vi "Heat Up Macro Find Small Flow Index.vi"(6 "Gallons":string[](array[string]), 8 "Error In":errorcluster, 9 "Draw Flag Column":string[](array[string]), 10 "Elapsed Time":string[](array[string]), 11 "Gallon Target":dbl) -> (0 "Error Out":errorcluster, 1 "Gallons":dbl, 2 "Time":dbl, 3 "Error Array. If all false":bool[](array[boolean]), 4 "Numeric":i32)   [LabVIEW 2019]
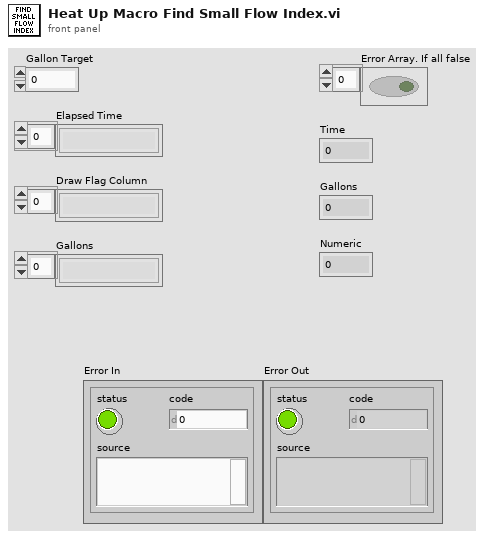
[diagram p1: front panel]
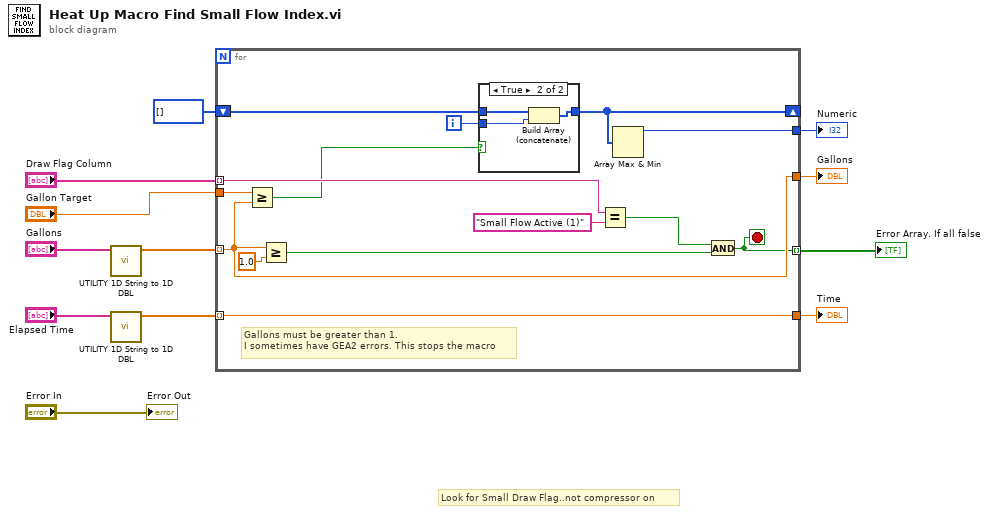
[diagram p0: block diagram]
diagram:
  # "Look for Small Draw Flag..not compressor on"
  n1 = call "UTILITY 1D String to 1D DBL.vi"("Save Data"="Gallons") -> ("DBL"=w3:dbl[])  [unwired: 10 in]
  n2 = call "UTILITY 1D String to 1D DBL.vi"("Save Data"="Elapsed Time") -> ("DBL"=w6:dbl[])  [unwired: 10 in]
  n3 = for {
    tunnel: w3 -> [w17] mode=indexing
    tunnel: [w17] -> w4
    tunnel: w6 -> [w26] mode=indexing
    tunnel: [w26] -> w9
    tunnel: "Gallon Target" -> [w25]
    shift-right: [w23] -> _
    shift-left: i32[] [] -> [w24]
    tunnel: [w22] -> w12
    tunnel: "Draw Flag Column" -> [w20] mode=indexing
    tunnel: [w13] -> w11 mode=indexing
    i -> [w21]
    stop <- w13 stop-if-true
    # "Gallons must be greater than 1.\nI sometimes have GEA2 errors. This stops the macro"
    n4 = Greater Or Equal?(x=w25, y=w17) -> (x >= y?=w18:bool)
    n5 = Greater Or Equal?(x=w17, y=1.0) -> (x >= y?=w14:bool)
    n6 = case shown="True" w18 {
      tunnel: w24 -> [w27 w30]
      tunnel: [w27 w29] -> w23
      tunnel: w21 -> [_ w28]
      frame False {
      }
      frame True {
        n7 = Build Array (concatenate)(w30, w28) -> (w29:i32[])
      }
    }
    n8 = Equal?(x=w20, y="Small Flow Active (1)") -> (x = y?=w15:bool)
    n9 = Array Max & Min(array=w23) -> (max value=w22:i32)  [unwired: 3 out]
    n10 = And(x=w15, y=w14) -> (x .and. y?=w13:bool)
  }
  "Numeric" <- w12
  "Error Array. If all false" <- w11
  "Time" <- w9
  "Gallons" <- w4
  "Error Out" <- "Error In"
